vi "WriteH5DataTest.vi"   [LabVIEW 2012]
uses:
  <vilib>/addons/h5labview2/file/H5Fmode.ctl
  <vilib>/Analysis/1siggen.llb/Ramp Pattern by Delta.vi
  <vilib>/addons/h5labview2/base/lib_path.vi
  <vilib>/addons/h5labview2/base/H5Equery.vi
  <vilib>/addons/h5labview2/attrib/H5Awrite.llb/H5Awrite.xnode
  <vilib>/addons/h5labview2/dataset/H5Dwrite.llb/H5Dwrite.xnode
  <vilib>/addons/h5labview2/file/H5F.lvlib
  <vilib>/addons/h5labview2/group/H5G.lvlib
  <vilib>/Analysis/NI_AALBase.lvlib
types:
  T1 = typedef "H5F.lvlib/H5Fmode.ctl" = enum16{"read-only", "read-write", "overwrite", "create new", "open or create"}
  T2 = typedef "hid_t.ctl" = i64
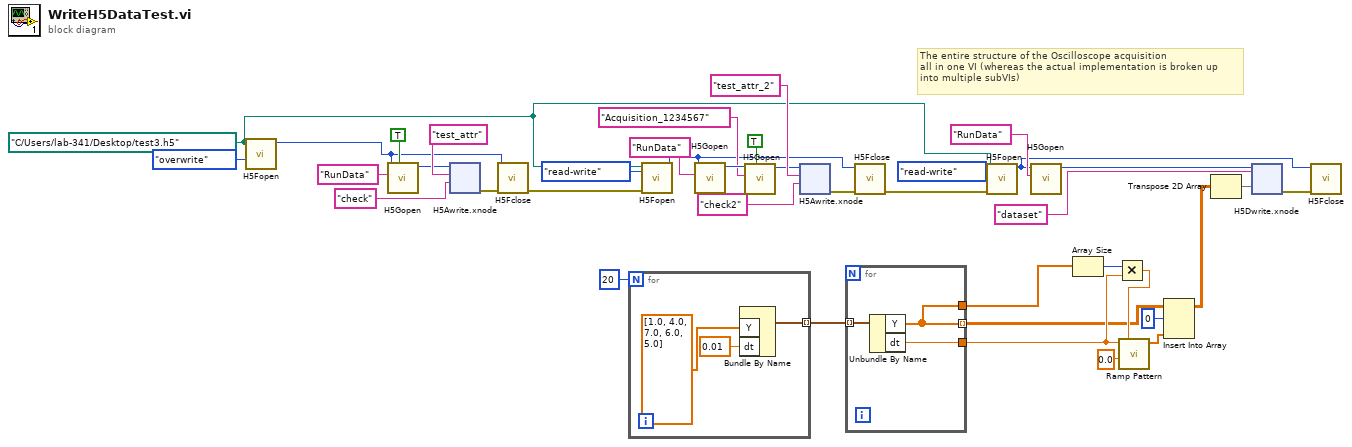
[diagram p0: block diagram]
diagram:
  w23 = path "C:/Users/lab-341/Desktop/test3.h5" ("path")
  # "The entire structure of the Oscilloscope acquisition\nall in one VI (whereas the actual implementation is broken up\ninto multiple subVIs)"
  n1 = call <vilib>:"H5Fopen.vi"("mode (read-only)"=H5Fmode."overwrite", "path"=w23) -> ("ref out"=w15:T2)  [unwired: 8 in, 1 out]
  n2 = call <vilib>:"H5Gopen.vi"("create? (F)"=TRUE, "name"="RunData", "ref in"=w15) -> ("group out"=w20:T2)  [unwired: 7 in, 1 out]
  n3 = xnode "H5Awrite.xnode"("data"="check" ("attrib name"), "attrib name"="test_attr", "ref in"=w20) -> ("error out"=w19:errorcluster)  [unwired: 4 in, 2 out]
  n4 = call <vilib>:"H5Fclose.vi"("error in (no error)"=w19, "ref"=w15) -> ("error out"=w31:errorcluster)  [unwired: 9 in]
  n5 = for {
    N: 20 -> [_]
    tunnel: [w42] -> w11 mode=indexing
    n6 = Bundle By Name("Y"=dbl[] [1.0, 4.0, 7.0, 6.0, 5.0], "dt"=0.01) -> (w42:waveform(dbl))  [unwired: 1 in]
  }
  n7 = call <vilib>:"H5Fopen.vi"("error in (no error)"=w31, "mode (read-only)"=H5Fmode."read-write", "path"=w23) -> ("ref out"=w14:T2)  [unwired: 7 in, 1 out]
  n8 = call <vilib>:"H5Gopen.vi"("name"="RunData", "ref in"=w14) -> ("group out"=w29:T2)  [unwired: 8 in, 1 out]
  n9 = call <vilib>:"H5Gopen.vi"("create? (F)"=TRUE, "name"="Acquisition_1234567", "ref in"=w29) -> ("group out"=w18:T2)  [unwired: 7 in, 1 out]
  n10 = xnode "H5Awrite.xnode"("data"="check2" ("attrib name"), "attrib name"="test_attr_2", "ref in"=w18) -> ("error out"=w17:errorcluster)  [unwired: 4 in, 2 out]
  n11 = for {
    tunnel: w11 -> [w45] mode=indexing
    tunnel: [w43] -> w3 mode=indexing
    tunnel: [w44] -> w4
    tunnel: [w43] -> w8
    n12 = Unbundle By Name(w45) -> ("Y"=w43:dbl[], "dt"=w44:dbl)
  }
  n13 = call <vilib>:"H5Fclose.vi"("error in (no error)"=w17, "ref"=w14) -> ("error out"=w24:errorcluster)  [unwired: 9 in]
  n14 = call <vilib>:"H5Fopen.vi"("error in (no error)"=w24, "mode (read-only)"=H5Fmode."read-write", "path"=w23) -> ("ref out"=w13:T2)  [unwired: 7 in, 1 out]
  n15 = call <vilib>:"H5Gopen.vi"("name"="RunData", "ref in"=w13) -> ("group out"=w12:T2)  [unwired: 8 in, 1 out]
  n16 = Array Size(array=w8) -> (size(s)=w9:i32)
  n17 = Multiply(x=w9, y=w4) -> (x*y=w7:dbl)
  n18 = call-poly <vilib>:"Ramp Pattern.vi"("start"=0.0, "end"=w7, "delta"=w4) -> ("Ramp Pattern"=w5:dbl[])  [unwired: 6 in, 2 out]
  n19 = Insert Into Array(array=w3, index (row)=0 ("index"), new element=w5) -> (w1:dbl[][])  [unwired: 1 in]
  n20 = Transpose 2D Array(2D array=w1) -> (transposed array=w2:dbl[][])
  n21 = xnode "H5Dwrite.xnode"("dataset name"="dataset", "data"=w2, "ref in"=w12) -> ("error out"=w16:errorcluster)  [unwired: 4 in, 2 out]
  n22 = call <vilib>:"H5Fclose.vi"("error in (no error)"=w16, "ref"=w13) -> ()  [unwired: 9 in, 1 out]
